vi "Insert Start Message.vi"(8 "error in (no error)":errorcluster, 10 "Start Time":timestamp, 11 "TrialBasedExperiment in":refnum<class "TrialBasedExperiment.lvclass">) -> (0 "error out":errorcluster, 3 "TrialBasedExperiment out":refnum<class "TrialBasedExperiment.lvclass">)   [LabVIEW 2010, in "TrialBasedExperiment.lvclass"]
uses:
  TrialBasedExperiment.lvclass
  Acquisition/Database/StimulationPrimary.ctl
  Acquisition/AcquistionObject/AcquistionObject.lvclass
  Acquisition/Database/SessionPrimary.ctl
  <vilib>/addons/database/NI_Database_API.lvlib
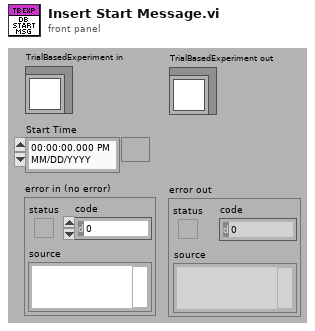
[diagram p1: front panel]
types:
  T1 = typedef "StimulationPrimary.ctl" = cluster{"setup":u8, "session_start_time":dbl, "stim_start_time":dbl}
  T2 = cluster{"setup":u8, "session_start_time":dbl, "stim_start_time":dbl, "stim_path":path, "exp_type":string}
  T3 = typedef "NI_Database_API.lvlib/Conn ObjectReference.ctl" = refnum<k1>
  T4 = typedef "SessionPrimary.ctl" = cluster{"setup":u8, "session_start_time":dbl}
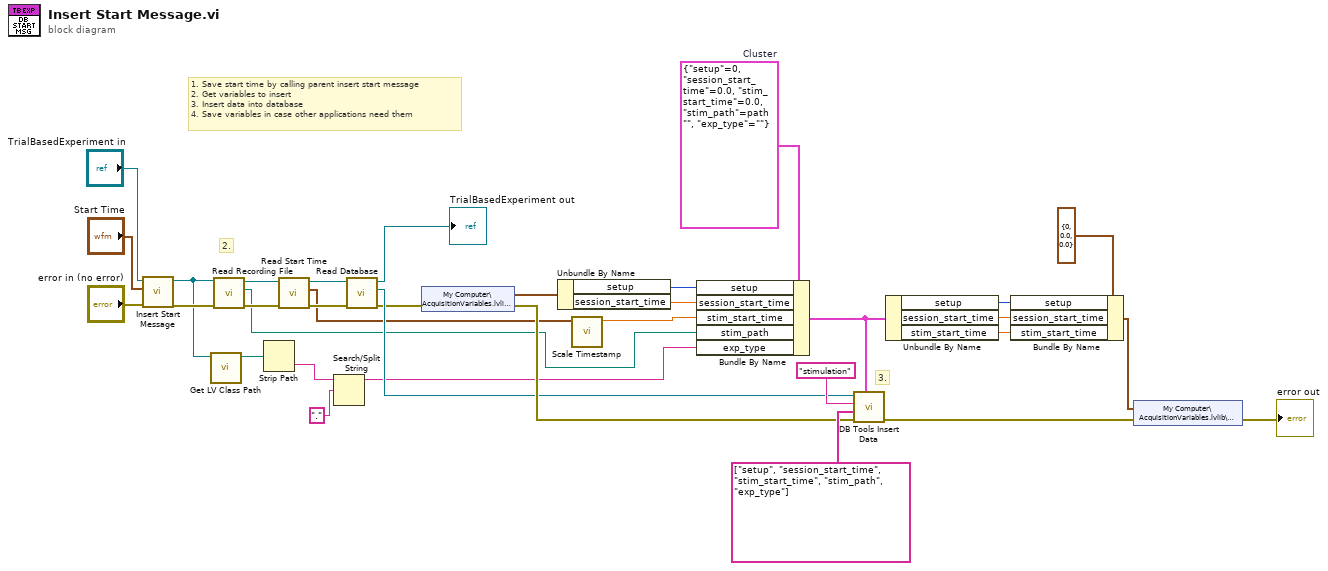
[diagram p0: block diagram]
diagram:
  w31 = T2 {"setup"=0, "session_start_time"=0.0, "stim_start_time"=0.0, "stim_path"=path "", "exp_type"=""}  # Cluster
  # "2."
  # "3."
  # "1. Save start time by calling parent insert start message\n2. Get variables to insert\n3. Insert data into database\n4. Save variables in case other applications need them"
  n1 = call-parent "Insert Start Message.vi"("error in (no error)"="error in (no error)", "Start Time"="Start Time", "AcquistionObject in"="TrialBasedExperiment in") -> ("error out"=w12:errorcluster, "AcquistionObject out"=w7:refnum<class "TrialBasedExperiment.lvclass">)  [unwired: 7 in]
  n2 = call <vilib>:"Get LV Class Path.vi"("object"=w7) -> ("class path"=w10:path)  [unwired: 9 in, 1 out]
  n3 = call-dynamic "Read Recording File.vi"("error in (no error)"=w12, "AcquistionObject in"=w7) -> ("error out"=w17:errorcluster, "Recording File"=w2:path, "AcquistionObject out"=w18:refnum<class "TrialBasedExperiment.lvclass">)  [unwired: 7 in]
  n4 = Strip Path(path=w10) -> (name=w9:string)  [unwired: 1 out]
  n5 = call-dynamic "Read Start Time.vi"("error in (no error)"=w17, "AcquistionObject in"=w18) -> ("error out"=w15:errorcluster, "Start Time"=w4:timestamp, "AcquistionObject out"=w16:refnum<class "TrialBasedExperiment.lvclass">)  [unwired: 7 in]
  n6 = Search/Split String(string=w9, search string/char (-)=".") -> (substring before match=w6:string)  [unwired: 1 in, 2 out]
  n7 = call-dynamic "Read Database.vi"("error in (no error)"=w15, "AcquistionObject in"=w16) -> ("error out"=w13:errorcluster, "reference"=w14:T3, "AcquistionObject out"=→"TrialBasedExperiment out":refnum<class "TrialBasedExperiment.lvclass">)  [unwired: 7 in]
  n8 = shared-variable "My Computer\\AcquisitionVariables.lvlib\\SessionPK"(error in=w13) -> (w22:T4, error out=w21:errorcluster)
  n9 = Unbundle By Name(w22) -> ("setup"=w28:u8, "session_start_time"=w27:dbl)
  n10 = call "Scale Timestamp.vi"("Time Stamp"=w4) -> ("Scaled timestamp"=w3:dbl)  [unwired: 10 in]
  n11 = Bundle By Name(cluster=w31, "setup"=w28, "session_start_time"=w27, "stim_start_time"=w3, "stim_path"=w2, "exp_type"=w6) -> (w26:T2)
  n12 = call <vilib>:"DB Tools Insert Data.vi"("data"=w26, "error in (no error)"=w21, "columns"=string[] ["setup", "session_start_time", "stim_start_time", "stim_path", "exp_type"], "table"="stimulation", "connection reference"=w14) -> ("error out"=w19:errorcluster)  [unwired: 5 in, 1 out]
  n13 = Unbundle By Name(w26) -> ("setup"=w25:u8, "session_start_time"=w24:dbl, "stim_start_time"=w23:dbl)
  n14 = Bundle By Name(cluster=T1 {"setup"=0, "session_start_time"=0.0, "stim_start_time"=0.0} ("StimulationPK"), "setup"=w25, "session_start_time"=w24, "stim_start_time"=w23) -> (w20:T1)
  n15 = shared-variable "My Computer\\AcquisitionVariables.lvlib\\StimulationPK"(w20, error in=w19) -> (error out=→"error out":errorcluster)
